vi "Create.vi"(8 "error in (no error)":errorcluster) -> (0 "error out":errorcluster, 3 "MultiErrors out":refnum<class "MultiErrors.lvclass">)   [LabVIEW 2020, in "Volatus.lvlib" / "MultiErrors.lvclass"]
uses:
  MultiErrors.lvclass
  MultiError Entry.ctl
  MultiErrors.lvclass/MultiErrors.ctl
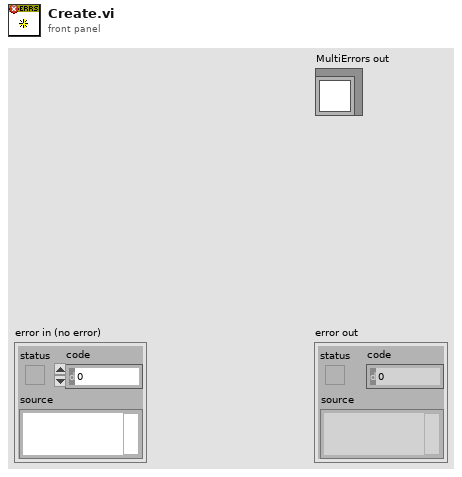
[diagram p1: front panel]
types:
  T1 = typedef "Volatus.lvlib/MultiErrors.lvclass/MultiError Entry.ctl" = cluster{"Context":string[], "Message":string, "Code":i32, "Call Chain":string[]}
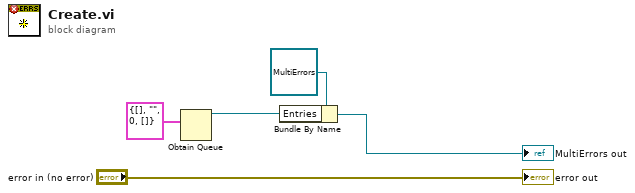
[diagram p0: block diagram]
diagram:
  n1 = Obtain Queue(element data type=T1 {"Context"=[], "Message"="", "Code"=0, "Call Chain"=[]} ("MultiError Entry")) -> (queue out=w1:refnum<queue>)  [unwired: 4 in, 2 out]
  n2 = Bundle By Name(cluster=refnum<class "MultiErrors.lvclass"> refnum ("MultiErrors in"), "Entries"=w1) -> (→"MultiErrors out":refnum<class "MultiErrors.lvclass">)
  "error out" <- "error in (no error)"
